vi "createWave.vi"(8 "error in (no error)":errorcluster, 10 "singleToneData":T1(array[cluster]), 11 "SoundDeviceData in":refnum<class "SoundDeviceData.lvclass">) -> (0 "error out":errorcluster, 1 "times":dbl[](array[numeric]), 2 "dataArray":dbl[][](array[numeric]), 3 "SoundDeviceData out":refnum<class "SoundDeviceData.lvclass">)   [LabVIEW 2009, in "DataMappers.lvlib" / "SoundDeviceData.lvclass"]
uses:
  SoundDeviceData.lvclass
  DatabaseHelpers/Database Objects/Channel/Channel.lvclass
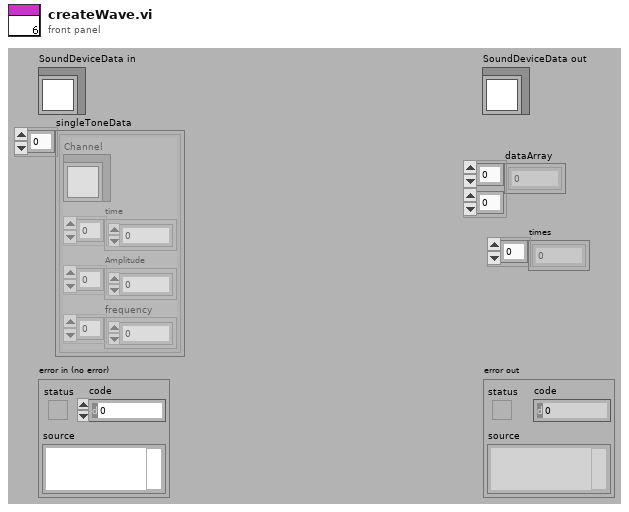
[diagram p1: front panel]
types:
  T1 = cluster{"Channel":refnum<class "Channel.lvclass">, "time":dbl[], "Amplitude":dbl[], "frequency":dbl[]}[]
  T2 = cluster{"Channel":refnum<class "Channel.lvclass">, "time":dbl[], "Amplitude":dbl[], "frequency":dbl[]}
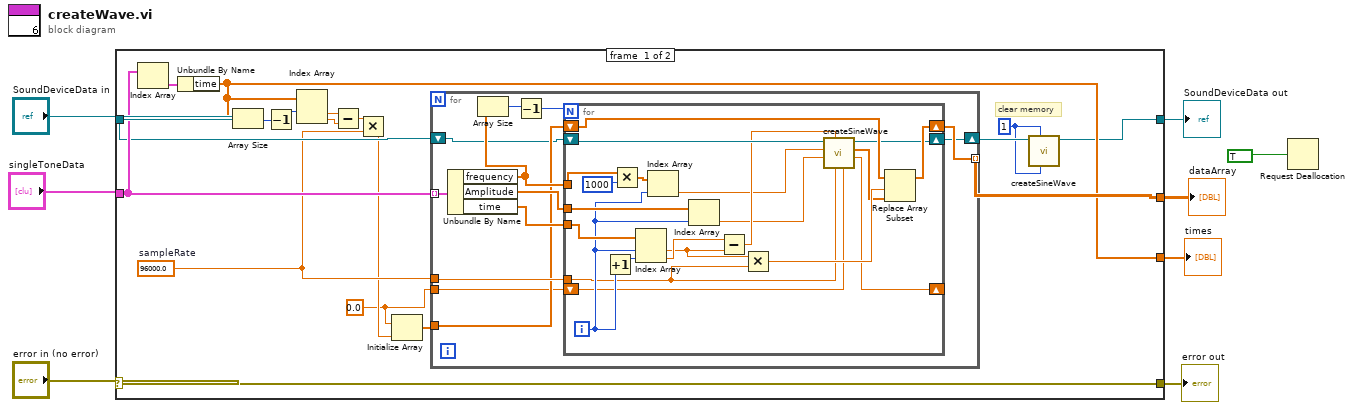
[diagram p0: block diagram]
diagram:
  n1 = case shown="No Error" "error in (no error)" {
    selector: "error in (no error)" -> [w26 w61]
    tunnel: [w26 w61] -> w7
    tunnel: [w10 w60] -> w5
    tunnel: "SoundDeviceData in" -> [w23 w60]
    tunnel: "singleToneData" -> [w25 _]
    tunnel: [w21 _] -> w3
    tunnel: [w22 _] -> w2
    frame #0 {
      w12 = 0.0
      w15 = 96000.0  # sampleRate
      w9 = 1
      # "clear memory"
      n2 = Index Array(array=w25) -> (element=w24:T2)  [unwired: 1 in]
      n3 = Unbundle By Name(w24) -> ("time"=w21:dbl[])
      n4 = Array Size(array=w21) -> (size(s)=w20:i32)
      n5 = Decrement(x=w20) -> (x-1=w19:i32)
      n6 = Index Array(array=w21, index #1=w19) -> (element #1=w17:dbl, element #2=w18:dbl)  [unwired: 1 in]
      n7 = Subtract(x=w17, y=w18) -> (x-y=w16:dbl)
      n8 = Multiply(x=w16, y=w15) -> (x*y=w13:dbl)
      n9 = Initialize Array(w12, w13) -> (w14:dbl[])
      n10 = for {
        tunnel: w25 -> [w38] mode=indexing
        tunnel: w15 -> [w37]
        tunnel: w14 -> [w31]
        tunnel: [w30] -> w22 mode=indexing
        shift-right: [w28] -> w11
        shift-left: w23 -> [w29]
        tunnel: w12 -> [w27]
        n11 = Unbundle By Name(w38) -> ("frequency"=w34:dbl[], "Amplitude"=w35:dbl[], "time"=w36:dbl[])
        n12 = Array Size(array=w34) -> (size(s)=w33:i32)
        n13 = Decrement(x=w33) -> (x-1=w32:i32)
        n14 = for {
          N: w32 -> [_]
          tunnel: w36 -> [w59]
          tunnel: w34 -> [w54]
          tunnel: w35 -> [w56]
          shift-right: [w50] -> w30
          shift-left: w31 -> [w51]
          tunnel: w37 -> [w45]
          shift-right: [w47] -> w28
          shift-left: w29 -> [w48]
          shift-right: [w39] -> _
          shift-left: w27 -> [w41]
          i -> [w52]
          n15 = Increment(x=w52) -> (x+1=w58:i32)
          n16 = Multiply(x=w54, y=1000) -> (x*y=w55:dbl[])
          n17 = Index Array(array=w59, index #1=w52, index #2=w58) -> (element #1=w44:dbl, element #2=w57:dbl)
          n18 = Index Array(array=w55, index=w52) -> (element=w43:dbl)
          n19 = Index Array(array=w56, index=w52) -> (element=w42:dbl)
          n20 = Subtract(x=w57, y=w44) -> (x-y=w46:dbl)
          n21 = Multiply(x=w44, y=w45) -> (x*y=w49:dbl)
          n22 = call "createSineWave.vi"("phase"=w41, "sampleRate"=w45, "duration"=w46, "Amplitude"=w42, "freq"=w43, "SoundDeviceData in"=w48) -> ("phase out"=w39:dbl, "sineWave"=w40:dbl[], "SoundDeviceData out"=w47:refnum<class "SoundDeviceData.lvclass">)  [unwired: 2 in, 1 out]
          n23 = Replace Array Subset(array=w51, new element=w40, index=w49) -> (w50:dbl[])
        }
      }
      n24 = call "createSineWave.vi"("sampleRate"=w9, "duration"=w9, "SoundDeviceData in"=w11) -> ("SoundDeviceData out"=w10:refnum<class "SoundDeviceData.lvclass">)  [unwired: 5 in, 3 out]
    }
    frame #1 {
    }
  }
  "error out" <- w7
  "SoundDeviceData out" <- w5
  "dataArray" <- w2
  "times" <- w3
  n25 = Request Deallocation(TRUE) -> ()
